vi "ttc.vi"(3 "x[k-1]":cluster{"v1":dbl, "v2":dbl, "SoC":dbl}, 4 "I":dbl, 5 "Period":u32=1000) -> (1 "model":T1 {"output"."Eeq" format="%#.6g"; "output"."Zeq" format="%#.6g"})   [LabVIEW 2021]
panel:
  in  "SOC":dbl[](array[numeric])=[0.0, 17.0, 27.0, 37.0, 47.0, 56.0, 67.0, 76.0, 88.0, 97.0, 100.0]
  in  "R0":dbl[](array[numeric])=[2.4, 1.25, 0.85, 0.7, 0.68, 0.67, 0.7, 0.83, 0.82, 0.82, 0.82]
  out "R0(SoC)":dbl format="%#.6g"
  in  "Em":dbl[](array[numeric])=[530.0, 542.0, 554.0, 564.0, 573.0, 582.0, 582.0, 612.0, 628.0, 630.0, 630.0]
  in  "R2":dbl[](array[numeric])=[0.15, 0.17, 0.19, 0.2, 0.19, 0.19, 0.2, 0.22, 0.22, 0.22, 0.22]
  in  "C2":dbl[](array[numeric])=[30.0, 24.0, 20.0, 19.0, 18.0, 15.0, 10.0, 5.0, 0.5, 1.0, 1.0]
  in  "R1":dbl[](array[numeric])=[1.9, 1.5, 1.5, 1.5, 1.5, 1.5, 1.4, 1.4, 1.4, 1.4, 1.4]
  out "tau1":dbl format="%#.6g"
  out "tau2":dbl format="%#.6g"
  out "Em(SoC)":dbl format="%#.6g"
  out "R2(SoC)":dbl format="%#.6g"
  out "C2(SoC)":dbl format="%#.6g"
  out "R1(SoC)":dbl format="%#.6g"
  out "C1(SoC)":dbl format="%#.6g"
  in  "C1":dbl[](array[numeric])=[300.0, 320.0, 350.0, 369.0, 368.0, 380.0, 382.0, 385.0, 386.0, 386.0, 386.0]
  # "LOOK-UP TABLE"
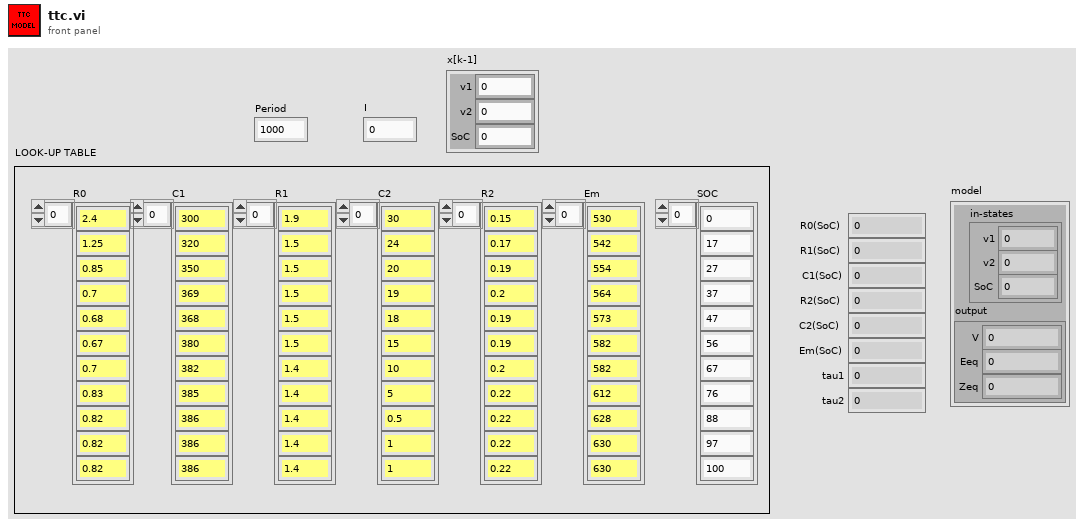
[diagram p1: front panel]
types:
  T1 = cluster{"in-states":cluster{"v1":dbl, "v2":dbl, "SoC":dbl}, "output":cluster{"V":dbl, "Zeq":dbl, "Eeq":dbl}}
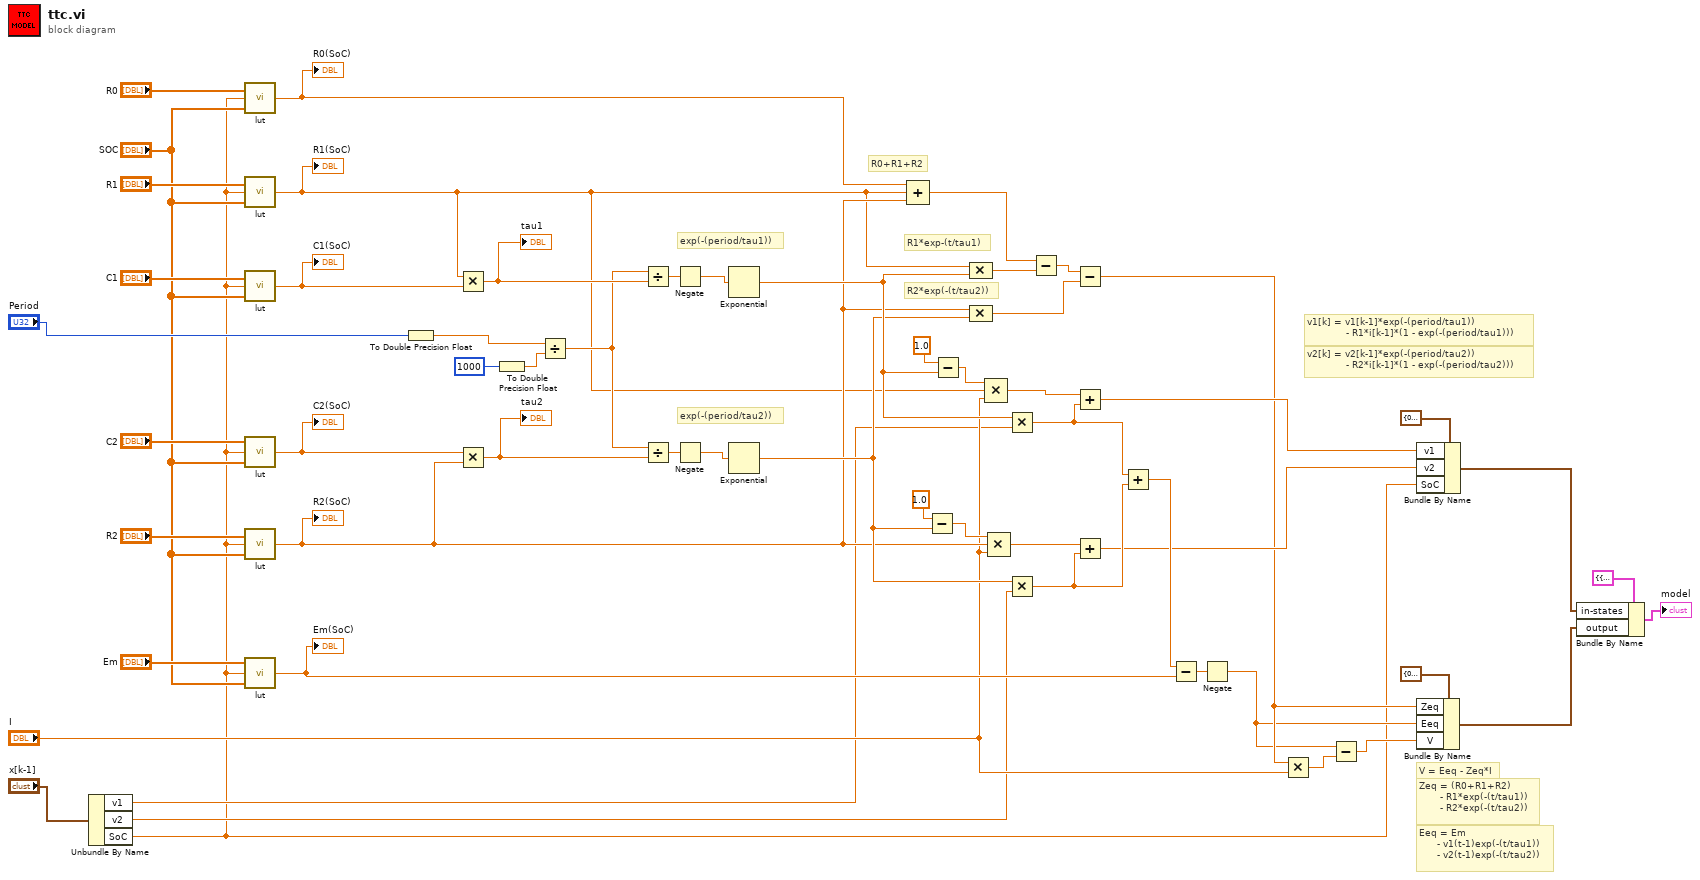
[diagram p0: block diagram]
diagram:
  # "V = Eeq - Zeq*I"
  # "v2[k] = v2[k-1]*exp(-(period/tau2))\n             - R2*i[k-1]*(1 - exp(-(period/tau2)))"
  # "v1[k] = v1[k-1]*exp(-(period/tau1))\n             - R1*i[k-1]*(1 - exp(-(period/tau1)))"
  # "Eeq = Em\n      - v1(t-1)exp(-(t/tau1))\n      - v2(t-1)exp(-(t/tau2))"
  # "R2*exp(-(t/tau2))"
  # "R1*exp-(t/tau1)"
  # "Zeq = (R0+R1+R2) \n       - R1*exp(-(t/tau1))\n       - R2*exp(-(t/tau2))"
  # "R0+R1+R2"
  # "exp(-(period/tau2))"
  # "exp(-(period/tau1))"
  n1 = Unbundle By Name("x[k-1]") -> ("v1"=w8:dbl, "v2"=w7:dbl, "SoC"=w3:dbl)
  n2 = call "lut.vi"("SOC"="SOC", "soc"=w3, "param"="R0") -> ("param(soc)"=w35:dbl)
  "R0(SoC)" <- w35
  n3 = call "lut.vi"("SOC"="SOC", "soc"=w3, "param"="R1") -> ("param(soc)"=w17:dbl)
  "R1(SoC)" <- w17
  n4 = call "lut.vi"("SOC"="SOC", "soc"=w3, "param"="C1") -> ("param(soc)"=w19:dbl)
  "C1(SoC)" <- w19
  n5 = call "lut.vi"("SOC"="SOC", "soc"=w3, "param"="C2") -> ("param(soc)"=w20:dbl)
  "C2(SoC)" <- w20
  n6 = call "lut.vi"("SOC"="SOC", "soc"=w3, "param"="R2") -> ("param(soc)"=w18:dbl)
  "R2(SoC)" <- w18
  n7 = call "lut.vi"("SOC"="SOC", "soc"=w3, "param"="Em") -> ("param(soc)"=w24:dbl)
  "Em(SoC)" <- w24
  n8 = To Double Precision Float(number="Period") -> (double precision float=w26:dbl)
  n9 = Multiply(x=w17, y=w19) -> (x*y=w54:dbl)
  "tau1" <- w54
  n10 = Multiply(x=w20, y=w18) -> (x*y=w36:dbl)
  "tau2" <- w36
  n11 = To Double Precision Float(number=i64 1000 ("y")) -> (double precision float=w25:dbl)
  n12 = Divide(x=w26, y=w25) -> (x/y=w48:dbl)
  n13 = Divide(x=w48, y=w54) -> (x/y=w55:dbl)
  n14 = Divide(x=w48, y=w36) -> (x/y=w53:dbl)
  n15 = Negate(x=w55) -> (-x=w57:dbl)
  n16 = Negate(x=w53) -> (-x=w56:dbl)
  n17 = Exponential(1:w57) -> (0:w37:dbl)
  n18 = Exponential(1:w56) -> (0:w30:dbl)
  n19 = Compound Arithmetic op=ADD(w35, w17, w18) -> (w46:dbl)
  n20 = Subtract(x=1.0, y=w30) -> (x-y=w34:dbl)
  n21 = Subtract(x=1.0, y=w37) -> (x-y=w33:dbl)
  n22 = Compound Arithmetic op=MULTIPLY(w17, w37) -> (w44:dbl)
  n23 = Compound Arithmetic op=MULTIPLY(w18, w30) -> (w32:dbl)
  n24 = Compound Arithmetic op=MULTIPLY(w33, w17, "I") -> (w31:dbl)
  n25 = Compound Arithmetic op=MULTIPLY(w34, w18, "I") -> (w50:dbl)
  n26 = Multiply(x=w37, y=w8) -> (x*y=w28:dbl)
  n27 = Multiply(x=w30, y=w7) -> (x*y=w29:dbl)
  n28 = Subtract(x=w46, y=w44) -> (x-y=w45:dbl)
  n29 = Subtract(x=w45, y=w32) -> (x-y=w12:dbl)
  n30 = Add(x=w31, y=w28) -> (x+y=w15:dbl)
  n31 = Add(x=w50, y=w29) -> (x+y=w14:dbl)
  n32 = Add(x=w28, y=w29) -> (x+y=w27:dbl)
  n33 = Subtract ("A")(x=w27, y=w24) -> (x-y=w49:dbl)
  n34 = Negate(x=w49) -> (-x=w10:dbl)
  n35 = Multiply(x=w12, y="I") -> (x*y=w23:dbl)
  n36 = Subtract(x=w10, y=w23) -> (x-y=w11:dbl)
  n37 = Bundle By Name(cluster=cluster{"v1":dbl, "v2":dbl, "SoC":dbl} {"v1"=0.0, "v2"=0.0, "SoC"=0.0} ("in-states"), "v1"=w15, "v2"=w14, "SoC"=w3) -> (w6:cluster{"v1":dbl, "v2":dbl, "SoC":dbl})
  n38 = Bundle By Name(cluster=cluster{"V":dbl, "Zeq":dbl, "Eeq":dbl} {"V"=0.0, "Zeq"=0.0, "Eeq"=0.0} ("y"), "Zeq"=w12, "Eeq"=w10, "V"=w11) -> (w5:cluster{"V":dbl, "Zeq":dbl, "Eeq":dbl})
  n39 = Bundle By Name(cluster=T1 {"in-states"={"v1"=0.0, "v2"=0.0, "SoC"=0.0}, "output"={"V"=0.0, "Zeq"=0.0, "Eeq"=0.0}} ("model"), "in-states"=w6, "output"=w5) -> (→"model":T1)
